vi "获取启动参数.vi"(7 "MB通信方式选择":enum16{"串口", "TCP"}(ring), 8 "Error in":errorcluster caption="Error in (no error)", 9 "Port (502)":u16=502, 10 "IP Address":string="localhost", 11 "VISA Resource":refnum<visa-resource-name>) -> (0 "error out":errorcluster, 3 "数组":cluster{"String":string, "Value":u16}[](array[cluster]))   [LabVIEW 2016, in "斯坦道CODCr.lvlib"]
uses:
  <vilib>/Plasmionique/MB Master/MB_Master_Serial/MB_Master_Serial.lvclass
  C:/Program Files (x86)/National Instruments/LabVIEW 2016/vi.lib/Plasmionique/MB Master/MB_Master/MB_Master.lvclass
  <vilib>/Plasmionique/MB Master/MB_Master_TCP/MB_Master_TCP.lvclass
  <vilib>/Plasmionique/MB Master/MB_Master/MB_Master.lvclass
  <vilib>/Plasmionique/MB Master/MB Master.lvlib
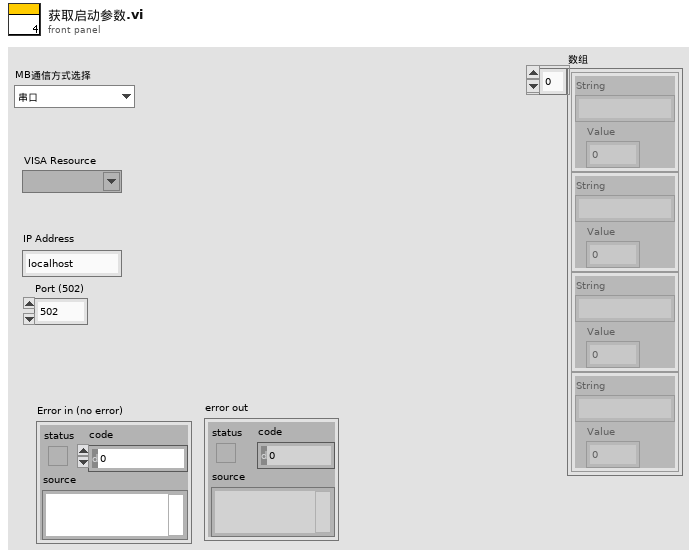
[diagram p1: front panel]
types:
  T1 = cluster{"baud rate (bps)":u32, "stop bits":u16, "parity":u16, "flow control":u16, "timeout":u32, "retries":i32}
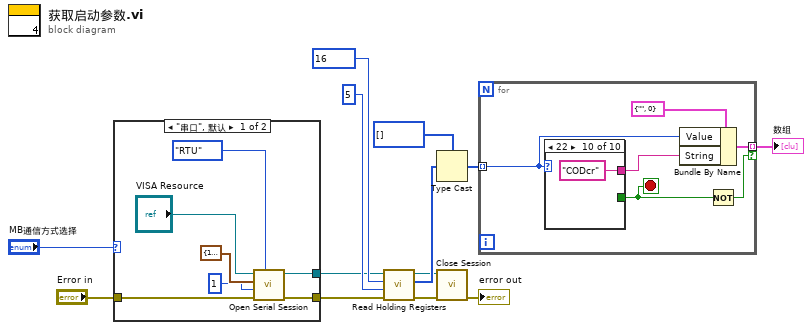
[diagram p0: block diagram]
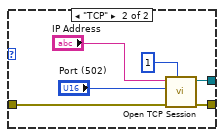
[diagram p2: hidden frame]
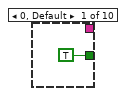
[diagram p3: hidden frame]
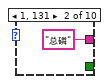
[diagram p4: hidden frame]
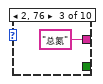
[diagram p5: hidden frame]
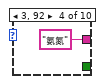
[diagram p6: hidden frame]
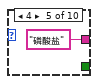
[diagram p7: hidden frame]
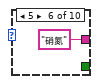
[diagram p8: hidden frame]
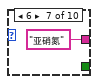
[diagram p9: hidden frame]
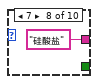
[diagram p10: hidden frame]
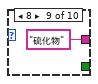
[diagram p11: hidden frame]
diagram:
  n1 = case shown="\"串口\", 默认" "MB通信方式选择" {
    tunnel: [w20 w26] -> w8
    tunnel: "Error in" -> [w15 w24]
    tunnel: [w14 w25] -> w4
    frame "串口", Default {
      n2 = call <vilib>:"Open Serial Session.vi"("Mode (RTU)"=enum16{"RTU", "ASCII"}."RTU", "Error in"=w15, "Slave ID"=u8 1, "Serial Config"=T1 {"baud rate (bps)"=115200, "stop bits"=10, "parity"=0, "flow control"=0, "timeout"=1000, "retries"=1}, "VISA Resource"="VISA Resource") -> ("Error out"=w14:errorcluster, "MB_Serial session"=w20:refnum<class "MB_Master_Serial.lvclass">)  [unwired: 5 in]
    }
    frame "TCP" {
      n3 = call <vilib>:"Open TCP Session.vi"("Slave ID (255)"=u8 1, "error in (no error)"=w24, "Port (502)"="Port (502)", "IP Address"="IP Address") -> ("error out"=w25:errorcluster, "MB_TCP session"=w26:refnum<class "MB_Master_TCP.lvclass">)  [unwired: 6 in]
    }
  }
  n4 = call <vilib>:"Read Holding Registers.vi"("error in (no error)"=w4, "quantity"=u16 5, "starting address"=u16 16, "MB session in"=w8) -> ("error out"=w3:errorcluster, "Registers"=w11:u16[], "MB session out"=w7:refnum<class "MB_Master.lvclass">)  [unwired: 5 in]
  n5 = Type Cast(type=u8[] [], x=w11) -> (*(type *) &x=w9:u8[])
  n6 = call-dynamic "Close Session.vi"("error in (no error)"=w3, "MB session in"=w7) -> ("error out"=→"error out":errorcluster)  [unwired: 9 in]
  n7 = for {
    tunnel: w9 -> [w29] mode=indexing
    tunnel: [w28] -> w6 mode=indexing if=w27
    stop <- w32 stop-if-true
    n8 = case shown="22" w29 {
      tunnel: [_ "总磷" ("table输入") "总氮" ("table输入") "氨氮" ("table输入") "磷酸盐" ("table输入") "硝氮" ("table输入") "亚硝氮" ("table输入") "硅酸盐" ("table输入") "硫化物" ("table输入") "CODcr" ("table输入")] -> w30
      tunnel: [TRUE _ _ _ _ _ _ _ _ _] -> w32
      frame 0, Default {
      }
      frame 1, 131 {
      }
      frame 2, 76 {
      }
      frame 3, 92 {
      }
      frame 4 {
      }
      frame 5 {
      }
      frame 6 {
      }
      frame 7 {
      }
      frame 8 {
      }
      frame 22 {
      }
    }
    n9 = Bundle By Name(cluster=cluster{"String":string, "Value":u16} {"String"="", "Value"=0}, "Value"=w29, "String"=w30) -> (w28:cluster{"String":string, "Value":u16})
    n10 = Not(x=w32) -> (.not. x?=w27:bool)
  }
  "数组" <- w6
